vi "pulse_generator.vi"(0 "Output Array":bool[](array[boolean])=[TRUE], 1 "Samples":i32=1, 2 "Low time (ms)":u32=80, 3 "High time (ms)":u32=20, 4 "Line(s)":tag="Dev2/port1/line0") -> ()   [LabVIEW 2017]
doc: "This example demonstrates how to generate digital output data using software timing.\n\nFor instructions on how to connect your signals from the DAQ device, refer to your device documentation."
uses:
  <vilib>/Utility/error.llb/DialogType.ctl
  <vilib>/DAQmx/write.llb/DAQmx Write (Digital 1D Bool 1Chan 1Samp).vi
  <vilib>/DAQmx/create/channels.llb/DAQmx Create Channel (DO-Digital Output).vi
  <vilib>/DAQmx/miscellaneous.llb/DAQmx Fill In Error Info.vi
panel:
  # "Channel Settings"
  # "Channel Settings"
  # "Data to Write"
  # "The number of enabled elements in the boolean array must equal the number of lines in the channel.\nTo disable an element: Right Click » Data Operations » Delete Element."
  # "Timing Settings"
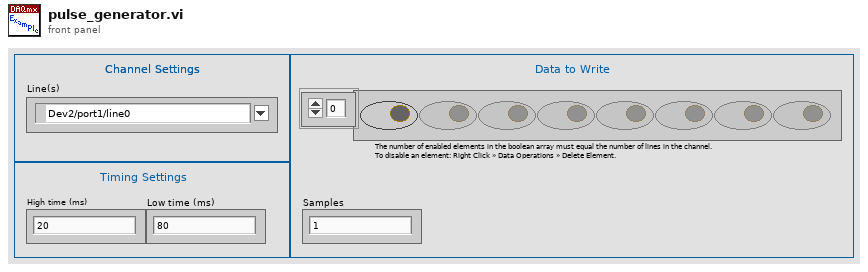
[diagram p1: front panel]
types:
  T1 = typedef "DialogType.ctl" = u16
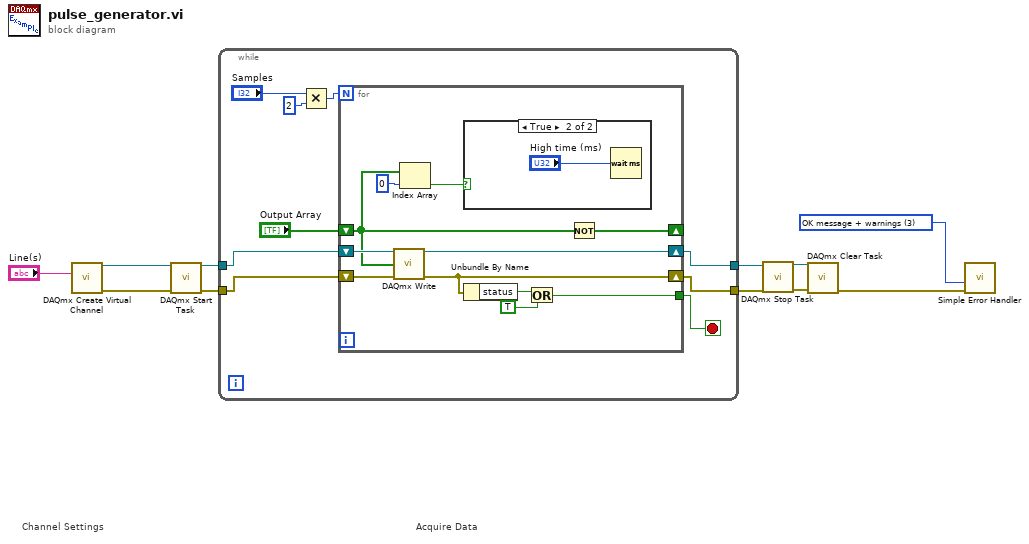
[diagram p0: block diagram]
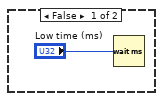
[diagram p2: hidden frame]
diagram:
  w1 = T1 3 items=["no dialog", "OK message", "continue or stop message", "OK message + warnings", "continue/stop + warnings"] ("type of dialog (OK msg:1)")
  # "Acquire Data"
  # "Channel Settings"
  n1 = call-poly <vilib>:"DAQmx Create Virtual Channel.vi"("lines"="Line(s)") -> ("task out"=w6:refnum<k21>, "error out"=w7:errorcluster)  [unwired: 13 in]
  n2 = call <vilib>:"DAQmx Start Task.vi"("task/channels in"=w6, "error in"=w7) -> ("task out"=w11:refnum<k21>, "error out"=w10:errorcluster)  [unwired: 12 in]
  n3 = while {
    tunnel: w11 -> [w20]
    tunnel: w10 -> [w19]
    tunnel: [w16] -> w2
    tunnel: [w17] -> w3
    stop <- w18 stop-if-true
    n4 = Multiply(x="Samples", y=2) -> (x*y=w15:i32)
    n5 = for {
      N: w15 -> [_]
      tunnel: [w29] -> w18
      shift-right: [w28] -> w17
      shift-left: w20 -> [w31]
      shift-right: [w27] -> w16
      shift-left: w19 -> [w30]
      shift-right: [w25] -> _
      shift-left: "Output Array" -> [w24]
      n6 = call-poly <vilib>:"DAQmx Write.vi"("task/channels in"=w31, "data"=w24, "error in"=w30) -> ("task out"=w28:refnum<k21>, "error out"=w27:errorcluster)  [unwired: 10 in, 1 out]
      n7 = Index Array(array=w24, index=0) -> (element=w22:bool)
      n8 = case shown="True" w22 {
        frame False {
          n9 = Wait (ms)(milliseconds to wait="Low time (ms)") -> ()  [unwired: 1 out]
        }
        frame True {
          n10 = Wait (ms)(milliseconds to wait="High time (ms)") -> ()  [unwired: 1 out]
        }
      }
      n11 = Unbundle By Name(w27) -> ("status"=w26:bool)
      n12 = Or(x=w26, y=TRUE) -> (x .or. y?=w29:bool)
      n13 = Not(x=w24) -> (.not. x?=w25:bool[])
    }
  }
  n14 = call <vilib>:"DAQmx Stop Task.vi"("task/channels in"=w3, "error in"=w2) -> ("task out"=w5:refnum<k21>, "error out"=w4:errorcluster)  [unwired: 12 in]
  n15 = call <vilib>:"DAQmx Clear Task.vi"("task in"=w5, "error in"=w4) -> ("error out"=w9:errorcluster)  [unwired: 13 in]
  n16 = call <vilib>:"Simple Error Handler.vi"("type of dialog (OK msg:1)"=w1, "error in (no error)"=w9) -> ()  [unwired: 3 in, 5 out]
